vi "Robot Global Data.vi"() -> ()   [LabVIEW 2012]
doc: "This global VI can contain as many global variables as you need. Place a control on the panel, give it a good name. To read or write to it from a VI, drag the icon to the diagram of that VI. You can also drag from the project. Click on the node to change which global you access. You shouldn't have multiple locations writing to a global or it will cause a race-condition."
uses:
  <vilib>/Rock Robotics/WPI/DriverStation/WPI_DriverStationRobotMode2.ctl
panel:
  out "Shooter Up":bool
  in  "Drive train right output":dbl
  in  "Drive train left output":dbl
  out "Right drive encoder dead":bool
  out "Left drive encoder dead":bool
  out "Vision Angle":dbl
  out "Shooter Encoder Dead":bool
  out "Shooter Ready":bool
  out "Shooter Speed":T1(ring)
  out "Came from disabled":bool
  out "Wheel Speed Info":T2(array[cluster])
  out "Debug Mode?":bool
  out "Hanging?":bool
  out "Reset Shooter PID":bool
  in  "Robot Mode":T3
  in  "LED toggle rate (ms)":u32=20
  # "Shooter"
  # "Asorted"
  # "Wheel Speed\n0 - DEFAULT/OFF\n1 - close 3pt\n2 - far 3pt\n3 - feeder shot\n4- upside down far 3pt\n\nno more at the moment"
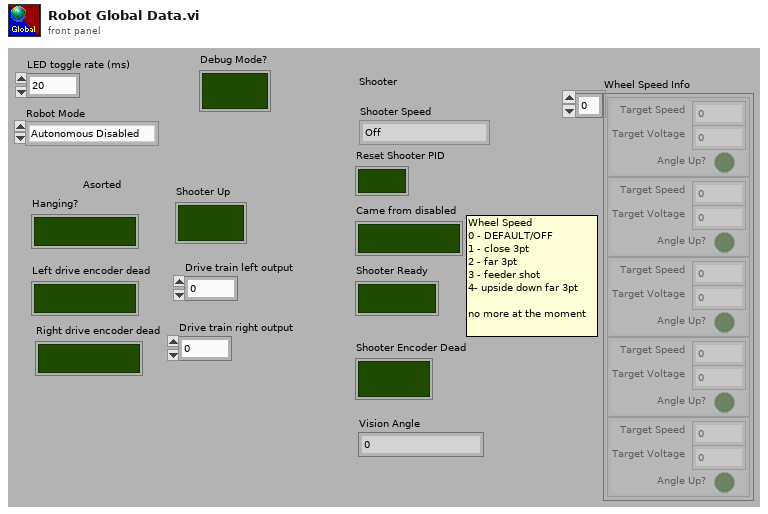
[diagram p1: front panel]
types:
  T1 = enum16{"Off", "Close Pyramid 3pt", "Far Pyramid 3pt", "Feeder Shot", "UD Far 3pt Shot"}
  T2 = cluster{"Target Voltage":dbl, "Target Speed":dbl, "Angle Up?":bool}[]
  T3 = typedef "WPI_DriverStationRobotMode2.ctl" = enum16{"Autonomous Disabled", "Autonomous Enabled", "Teleop Disabled", "Teleop Enabled", "Timeout", "Finish", "Test Disabled", "Test Enabled"}
diagram:
